vi "Layers To Decorate.vi"(9 "Actor To Decorate":refnum<class "Actor.lvclass">, 10 "Layers":refnum<class "Actor.lvclass">[](array[class])) -> (1 "Local Msg Sets":T1[](array[typedef]), 2 "Decorated Actor":refnum<class "Actor.lvclass">)   [LabVIEW 2025, in "jettl.lvlib"]
uses:
  jettl.lvlib
  Actor/Actor.lvclass
  Msg Set.ctl
  Msg/Msg.lvclass
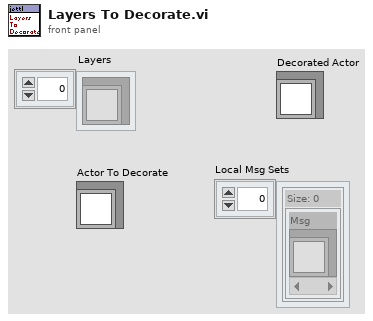
[diagram p1: front panel]
types:
  T1 = typedef "jettl.lvlib/Msg Set.ctl" = set{refnum<class "Msg.lvclass">}
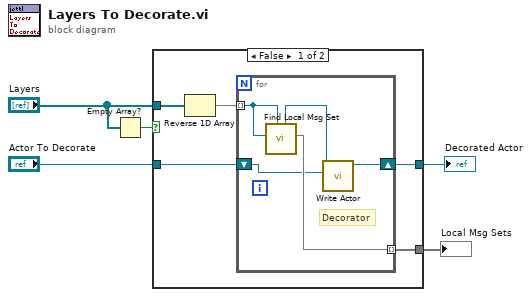
[diagram p0: block diagram]
diagram:
  n1 = Empty Array?(array="Layers") -> (empty?=w2:bool)
  n2 = case shown="False" w2 {
    tunnel: "Actor To Decorate" -> [w9 w16]
    tunnel: [w8 w16] -> w4
    tunnel: "Layers" -> [w7 _]
    tunnel: [w6 _] -> w1
    frame False {
      n3 = Reverse 1D Array(array=w7) -> (reversed array=w10:refnum<class "Actor.lvclass">[])
      n4 = for {
        tunnel: w10 -> [w15] mode=indexing
        shift-right: [w11] -> w8
        shift-left: w9 -> [w12]
        tunnel: [w14] -> w6 mode=indexing
        # "Decorator"
        n5 = call "Find Local Msg Set.vi"("Actor in"=w15, "X Actor.lvclass"=w15) -> ("Local Msg Set"=w14:T1, "Actor out"=w13:refnum<class "Actor.lvclass">)  [unwired: 8 in]
        n6 = call-dynamic "Write Actor.vi"("Actor"=w12, "Actor in"=w13) -> ("Actor out"=w11:refnum<class "Actor.lvclass">)  [unwired: 9 in]
      }
    }
    frame True {
    }
  }
  "Decorated Actor" <- w4
  "Local Msg Sets" <- w1
